vi "Begin.vi"() -> (0 "error out":errorcluster)   [LabVIEW 2013]
doc: "Called before other user functions, this VI is expected to open initial I/O refnums, load in file data, and do all program initialization. Notice that the <B>error out</B> terminal is simply used for data flow. Wiring it to other structures or subVIs ensures that this VI runs first."
uses:
  <vilib>/Rock Robotics/WPI/Joystick/WPI_JoystickDeviceEnum.ctl
  <vilib>/Rock Robotics/SystemInterfaces/Typedef/FPGA_TypedefDigitalModule.ctl
  <vilib>/Rock Robotics/SystemInterfaces/DIO/FPGA_DIOChannel.ctl
  <vilib>/Rock Robotics/SystemInterfaces/DIO/FPGA_DIORelayChannel.ctl
  <vilib>/Rock Robotics/SystemInterfaces/Typedef/FPGA_TypedefSolenoidModule.ctl
  <vilib>/Rock Robotics/WPI/Solenoid/WPI_SolenoidChannel.ctl
  <vilib>/Rock Robotics/WPI/Solenoid/WPI_SolenoidValue.ctl
  <vilib>/Rock Robotics/SystemInterfaces/DIO/FPGA_DIOPWMChannel.ctl
  <vilib>/Rock Robotics/WPI/Encoder/WPI_EncoderType.ctl
  <vilib>/Rock Robotics/WPI/Solenoid/WPI_SolenoidOpenDouble.vi
  <vilib>/Rock Robotics/WPI/Solenoid/WPI_SolenoidSetEnum.vi
  <vilib>/Rock Robotics/WPI/Counter/WPI_CounterDigitalInputToDigitalSource.vi
  <vilib>/Rock Robotics/WPI/RobotDrive/WPI_RobotDriveOpen2MotorWithVictor.vi
  <vilib>/Rock Robotics/WPI/MotorControl/WPI_MotorControlOpen Victor.vi
  <vilib>/Rock Robotics/WPI/Compressor/WPI_CompressorGetSetRefNum.vi
  <vilib>/Rock Robotics/WPI/Camera/WPI_CameraImageSize.ctl
  <vilib>/Rock Robotics/WPI/Camera/WPI_CameraWhite Balance Values.ctl
  <vilib>/Rock Robotics/WPI/Camera/WPI_CameraExposure Values.ctl
  <vilib>/Rock Robotics/WPI/Camera/WPI_CameraFrameRate.ctl
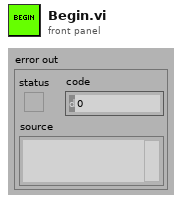
[diagram p1: front panel]
types:
  T1 = typedef "FPGA_DIOChannel.ctl" = enum8{"DIO 1", "DIO 2", "DIO 3", "DIO 4", "DIO 5", "DIO 6", "DIO 7", "DIO 8", "DIO 9", "DIO 10", "DIO 11", "DIO 12", "DIO 13", "DIO 14", "Invalid"}
  T2 = typedef "WPI_SolenoidChannel.ctl" = enum8{"Solenoid 1", "Solenoid 2", "Solenoid 3", "Solenoid 4", "Solenoid 5", "Solenoid 6", "Solenoid 7", "Solenoid 8", "Invalid"}
  T3 = typedef "FPGA_DIOPWMChannel.ctl" = enum8{"PWM 1", "PWM 2", "PWM 3", "PWM 4", "PWM 5", "PWM 6", "PWM 7", "PWM 8", "PWM 9", "PWM 10", "Invalid"}
  T4 = typedef "WPI_EncoderType.ctl" = enum16{"1x", "2x", "4x"}
  T5 = typedef "WPI_SolenoidValue.ctl" = enum16{"Off", "On", "Forward", "Reverse"}
  T6 = typedef "FPGA_TypedefSolenoidModule.ctl" = enum16{"Solenoid Module 1", "Solenoid Module 2"}
  T7 = typedef "FPGA_DIORelayChannel.ctl" = enum8{"Relay 1", "Relay 2", "Relay 3", "Relay 4", "Relay 5", "Relay 6", "Relay 7", "Relay 8", "Invalid"}
  T8 = typedef "WPI_JoystickDeviceEnum.ctl" = enum16{"USB 1", "USB 2", "USB 3", "USB 4", "Kinect 1", "Kinect 2"}
  T9 = typedef "FPGA_TypedefDigitalModule.ctl" = enum16{"Digital Module 1", "Digital Module 2"}
  T10 = typedef "WPI_CameraFrameRate.ctl" = u32
  T11 = typedef "WPI_CameraExposure Values.ctl" = enum16{"Auto", "Flicker-free 50 Hz", "Flicker-free 60 Hz", "Hold current"}
  T12 = typedef "WPI_CameraWhite Balance Values.ctl" = enum16{"Auto", "Fixed indoor", "Fixed outdoor 1", "Fixed outdoor 2", "Fixed fluorescent 1", "Fixed fluorescent 2", "Hold current"}
  T13 = typedef "WPI_CameraImageSize.ctl" = enum16{"640x480", "320x240", "160x120"}
  T14 = typedef "WPI_CameraDevRef.ctl" = cluster{"Camera Address":string, "CameraStatus":errorcluster, "Acquire Image Notifier":refnum<notifier>}
  T15 = typedef "WPI_DigitalInputDevRef.ctl" = cluster{"DevStatus":errorcluster, "DIO Channel":T1, "Digital Module":T9}
  T16 = typedef "WPI_MotorControlDeviceRef.ctl" = cluster{"DeviceStatus":errorcluster, "Type":enum16{"PWM", "CAN"}, "PWM":cluster{"Digital Module":T9, "PWM Channel":T3, "DeadBand":T17}, "CAN":cluster{"Device Number":u8, "Control Mode":T18, "Semaphore":T19, "Max Vout":dbl}, "Invert":bool, "TransformRef":T20, "InvTransformRef":T20}
  T17 = typedef "WPI_PWMDeadband.ctl" = cluster{"Name":string, "maxPositivePwm":i32, "minPositivePwm":i32, "centerPwm":i32, "maxNegativePwm":i32, "minNegativePwm":i32, "angularRange":u16}
  T18 = typedef "WPI_CANJaguar_ControlMode.ctl" = enum8{"Percent VBus", "Current", "Speed", "Position", "Voltage"}
  T19 = typedef "Semaphore RefNum" = refnum<k1>
  T20 = typedef "WPI_PWMTransform_ConPane.ctl" = refnum<vi>
  T21 = typedef "WPI_SolenoidDevRef.ctl" = cluster{"DevStatus":errorcluster, "Solenoid Module":T6, "Forward Solenoid Channel":T2, "Reverse Solenoid Channel":T2}
  T22 = typedef "FPGA_CounterEncoderSourceConvertionLVSourceType.ctl" = cluster{"DevStatus":errorcluster, "AnalogTriggerMode?":bool, "DigitalMode":cluster{"Digital Module":T9, "DIO Channel":T23}, "AnalogTriggerMode":cluster{"AnalogTriggerIndex":T24, "OutputType":T25}}
  T23 = typedef "FPGA_DIODigitalSourceChannel.ctl" = enum8{"DIO 1", "DIO 2", "DIO 3", "DIO 4", "DIO 5", "DIO 6", "DIO 7", "DIO 8", "DIO 9", "DIO 10", "DIO 11", "DIO 12", "DIO 13", "DIO 14", "Disabled"}
  T24 = typedef "FPGA_AnalogTriggerIndex.ctl" = enum8{"Trig 0", "Trig 1", "Trig 2", "Trig 3", "Trig 4", "Trig 5", "Trig 6", "Trig 7", "Invalid"}
  T25 = typedef "FPGA_AnalogTriggerOutType.ctl" = enum16{"InWindow", "TriggerState", "Rising", "Falling"}
  T26 = typedef "WPI_CompressorDevRef.ctl" = cluster{"DevStatus":errorcluster, "DigitalInputDevRef":T15, "RelayDevRef":T27}
  T27 = typedef "WPI_RelayDevRef.ctl" = cluster{"DevStatus":errorcluster, "Relay Channel":T7, "Digital Module":T9, "Relay Direction":T28}
  T28 = typedef "WPI_RelayDirection.ctl" = enum16{"Both directions", "Forward only", "Reverse only"}
  T29 = typedef "WPI_RobotDriveDevRef.ctl" = cluster{"DevStatus":errorcluster, "Motors[]":T16[], "Square Inputs":bool, "Max Output":dbl, "Isochronous":bool}
  T30 = typedef "WPI_EncoderDevRef.ctl" = cluster{"DevStatus":errorcluster, "EncoderIndex":T31, "CounterIndex":T32, "DistancePerCount":dbl, "Decoding Type":T4}
  T31 = typedef "FPGA_EncoderIdx.ctl" = enum8{"Enc 0", "Enc 1", "Enc 2", "Enc 3", "Invalid"}
  T32 = typedef "FPGA_CounterCtrSystemIndex.ctl" = enum8{"Ctr 0", "Ctr 1", "Ctr 2", "Ctr 3", "Ctr 4", "Ctr 5", "Ctr 6", "Ctr 7", "Invalid"}
  T33 = typedef "WPI_JoystickDevRef.ctl" = cluster{"Device":T8}
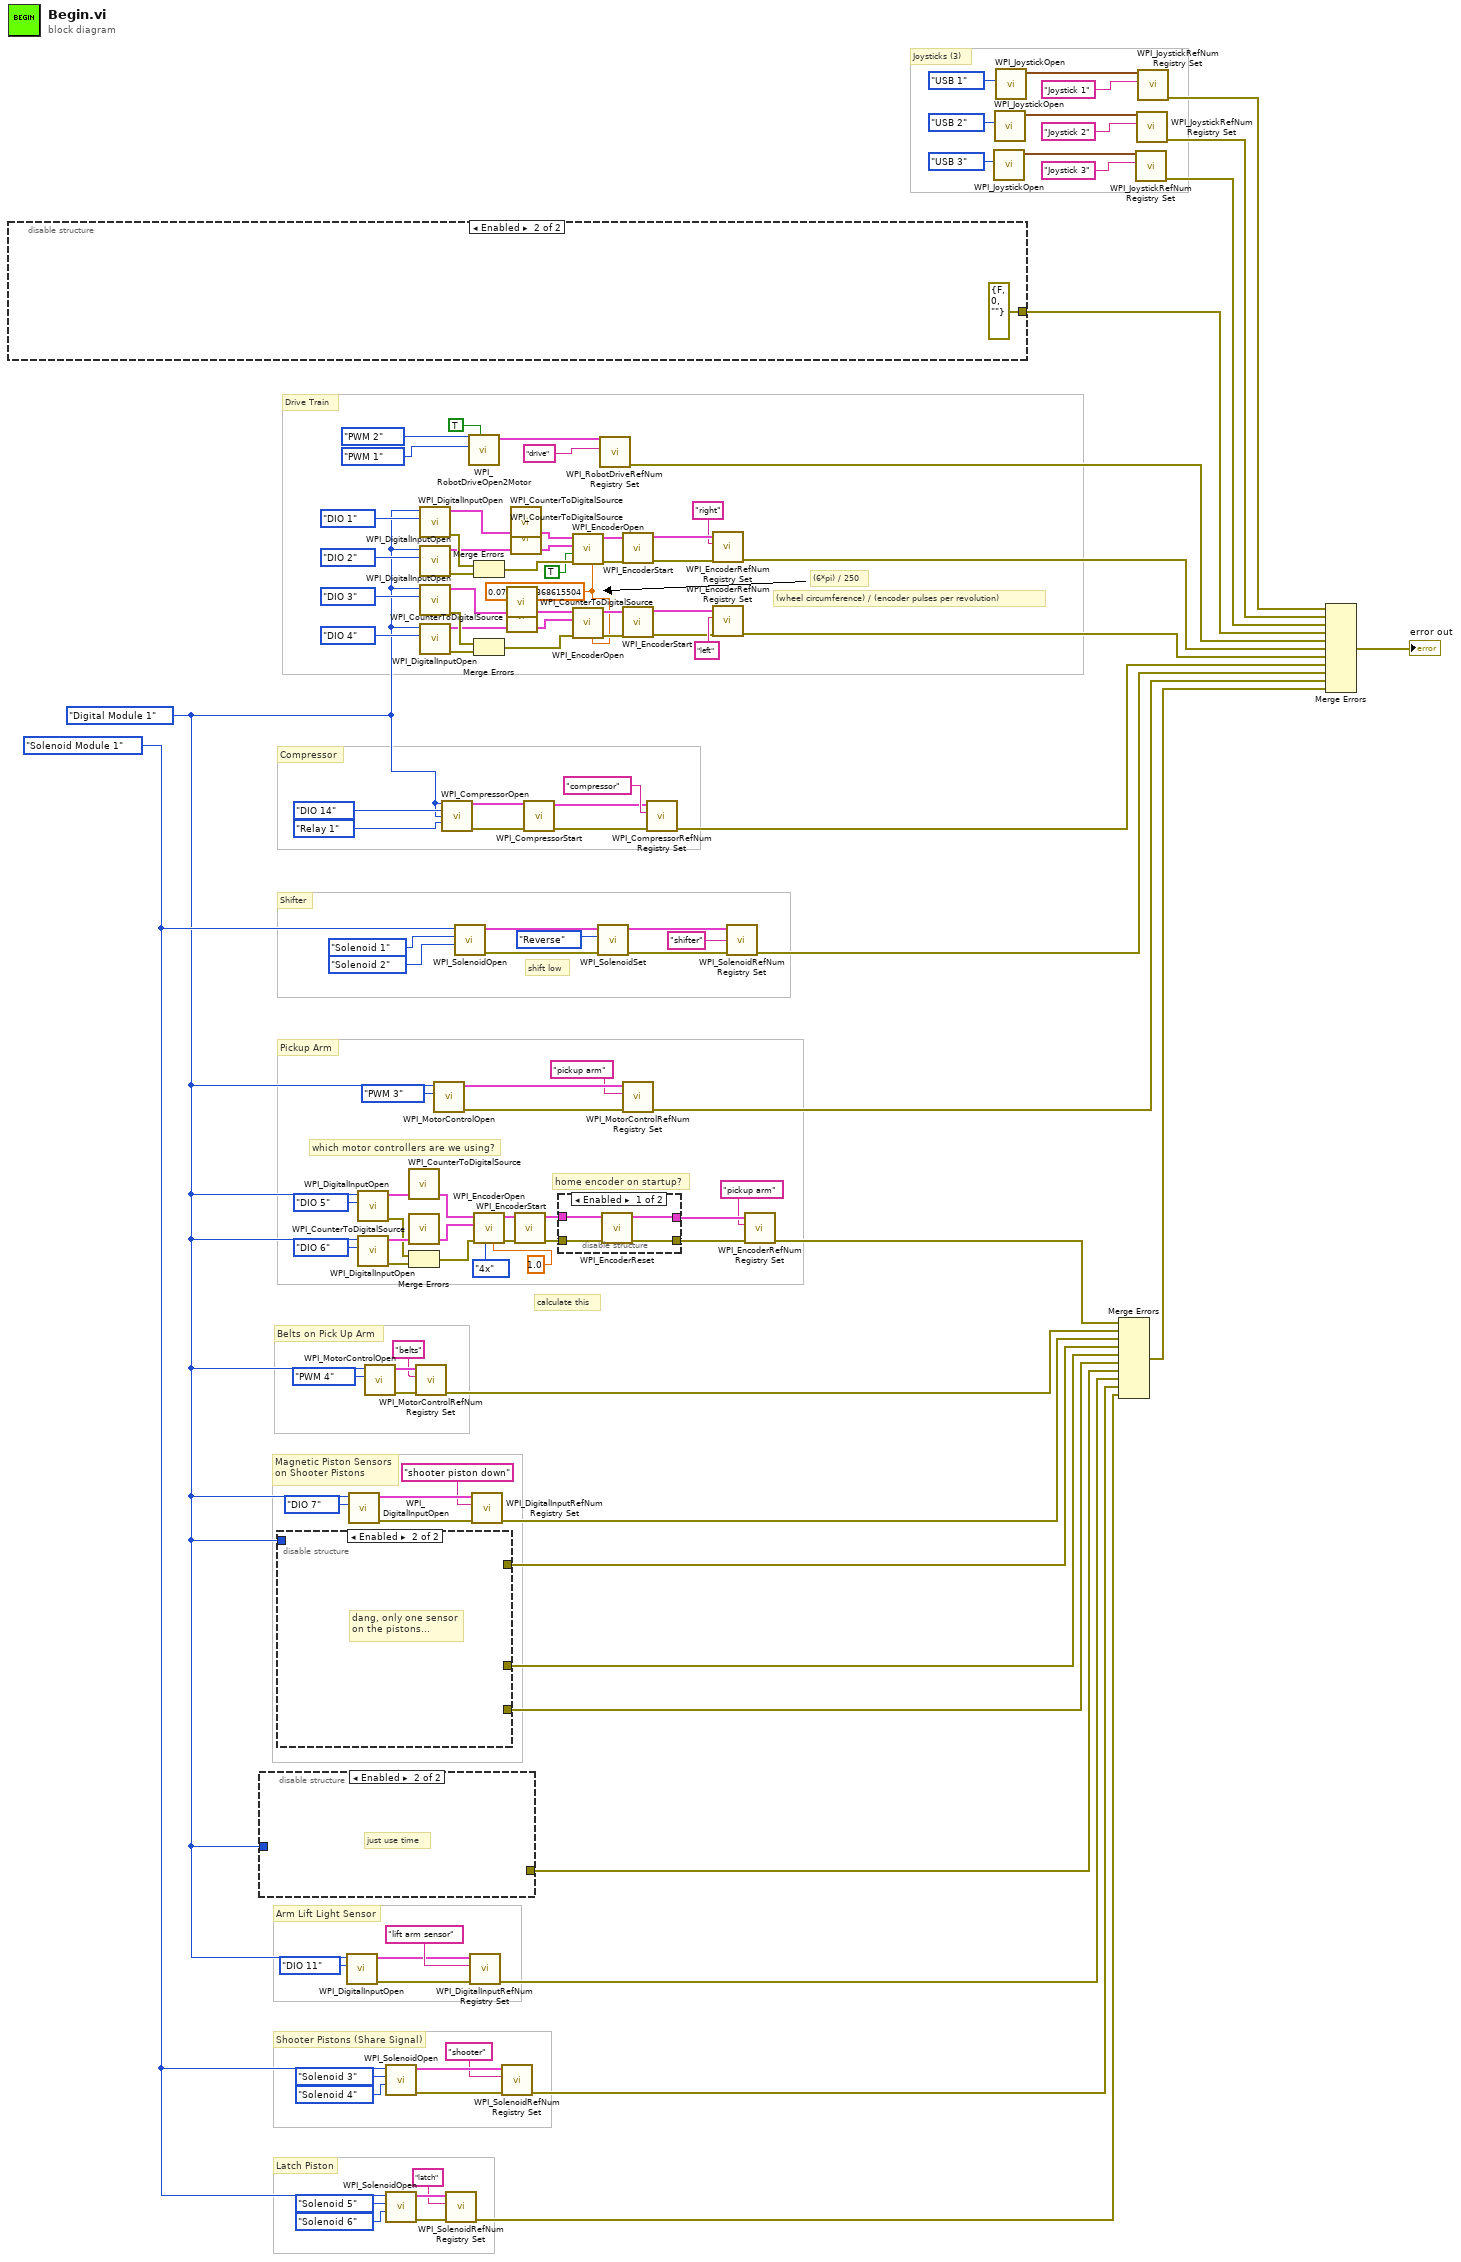
[diagram p0: block diagram]
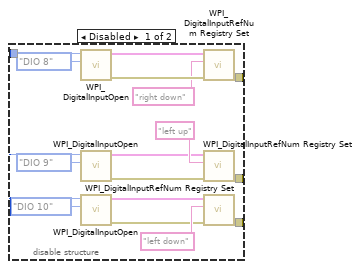
[diagram p2: hidden frame]
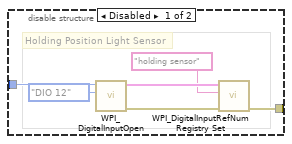
[diagram p3: hidden frame]
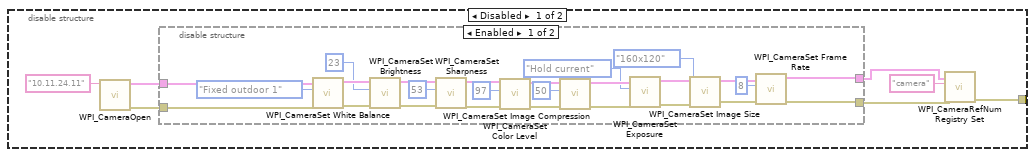
[diagram p5: hidden frame]
diagram:
  w71 = 0.07539822368615504 ("DistancePerCount")
  w12 = FPGA_TypedefSolenoidModule."Solenoid Module 1" ("Solenoid Module (Module 1)")
  w7 = FPGA_TypedefDigitalModule."Digital Module 1" ("Digital Module (Module 1)")
  # "Arm Lift Light Sensor"
  # "Joysticks (3)"
  # "Latch Piston"
  # "Shooter Pistons (Share Signal)"
  # "Magnetic Piston Sensors\non Shooter Pistons"
  # "Belts on Pick Up Arm"
  # "calculate this"
  # "Pickup Arm"
  # "home encoder on startup?"
  # "Shifter"
  # "Compressor"
  # "Drive Train"
  # "which motor controllers are we using?"
  # "shift low"
  # "(wheel circumference) / (encoder pulses per revolution)"
  # "(6*pi) / 250"
  n1 = disable-structure shown="Enabled" {
    disable-tunnel: [w128 errorcluster {"status"=FALSE, "code"=0, "source"=""} ("error out")] -> w115
    frame Disabled {
      n2 = call <vilib>:"WPI_CameraOpen.vi"("Camera Address"="10.11.24.11") -> ("error out"=w130:errorcluster, "CameraDevRef"=w132:T14)  [unwired: 9 in]
      n3 = disable-structure shown="Enabled" {
        disable-tunnel: w132 -> [w158 w162]
        disable-tunnel: [w136 w162] -> w131
        disable-tunnel: w130 -> [w145 w161]
        disable-tunnel: [w135 w161] -> w129
        frame Enabled {
          n4 = call <vilib>:"WPI_CameraSet White Balance.vi"("error in (no error)"=w145, "White Balance"=WPI_CameraWhite_Balance_Values."Fixed outdoor 1", "CameraDevRef"=w158) -> ("error out"=w146:errorcluster, "CameraDevRef Out"=w157:T14)  [unwired: 7 in]
          n5 = call <vilib>:"WPI_CameraSet Brightness.vi"("error in (no error)"=w146, "Brightness"=23, "CameraDevRef"=w157) -> ("error out"=w147:errorcluster, "CameraDevRef Out"=w156:T14)  [unwired: 7 in]
          n6 = call <vilib>:"WPI_CameraSet Sharpness.vi"("error in (no error)"=w147, "Sharpness"=53, "CameraDevRef"=w156) -> ("error out"=w148:errorcluster, "CameraDevRef Out"=w155:T14)  [unwired: 7 in]
          n7 = call <vilib>:"WPI_CameraSet Color Level.vi"("error in (no error)"=w148, "Color Level"=97, "CameraDevRef"=w155) -> ("error out"=w149:errorcluster, "CameraDevRef Out"=w154:T14)  [unwired: 7 in]
          n8 = call <vilib>:"WPI_CameraSet Image Compression.vi"("error in (no error)"=w149, "Compression"=50, "CameraDevRef"=w154) -> ("error out"=w160:errorcluster, "CameraDevRef Out"=w159:T14)  [unwired: 7 in]
          n9 = call <vilib>:"WPI_CameraSet Exposure.vi"("error in (no error)"=w160, "Exposure"=WPI_CameraExposure_Values."Hold current", "CameraDevRef"=w159) -> ("error out"=w150:errorcluster, "CameraDevRef Out"=w153:T14)  [unwired: 7 in]
          n10 = call <vilib>:"WPI_CameraSet Image Size.vi"("error in (no error)"=w150, "Image Size"=WPI_CameraImageSize."160x120", "CameraDevRef"=w153) -> ("error out"=w151:errorcluster, "CameraDevRef Out"=w152:T14)  [unwired: 7 in]
          n11 = call <vilib>:"WPI_CameraSet Frame Rate.vi"("error in (no error)"=w151, "Frame Rate (fps)"=T10 8, "CameraDevRef"=w152) -> ("error out"=w135:errorcluster, "CameraDevRef Out"=w136:T14)  [unwired: 7 in]
        }
        frame Disabled {
        }
      }
      n12 = call <vilib>:"WPI_CameraRefNum Registry Set.vi"("error in (no error)"=w129, "refnum name"="camera", "CameraDevRef"=w131) -> ("error out"=w128:errorcluster)  [unwired: 7 in, 1 out]
    }
    frame Enabled {
    }
  }
  n13 = disable-structure shown="Enabled" {
    disable-tunnel: w7 -> [w165 _]
    disable-tunnel: [w164 _] -> w3
    frame Disabled {
      # "Holding Position Light Sensor"
      n14 = call <vilib>:"WPI_DigitalInputOpen.vi"("DIO Channel"=FPGA_DIOChannel."DIO 12", "Digital Module (Module 1)"=w165) -> ("error out"=w168:errorcluster, "DigitalInputDevRef"=w167:T15)  [unwired: 8 in]
      n15 = call <vilib>:"WPI_DigitalInputRefNum Registry Set.vi"("error in (no error)"=w168, "refnum name"="holding sensor", "DigitalInputDevRef"=w167) -> ("error out"=w164:errorcluster)  [unwired: 7 in, 1 out]
    }
    frame Enabled {
      # "just use time"
    }
  }
  n16 = disable-structure shown="Enabled" {
    disable-tunnel: [w182 _] -> w23
    disable-tunnel: w7 -> [w172 _]
    disable-tunnel: [w171 _] -> w2
    disable-tunnel: [w170 _] -> w1
    frame Disabled {
      n17 = call <vilib>:"WPI_DigitalInputOpen.vi"("DIO Channel"=FPGA_DIOChannel."DIO 8", "Digital Module (Module 1)"=w172) -> ("error out"=w185:errorcluster, "DigitalInputDevRef"=w184:T15)  [unwired: 8 in]
      n18 = call <vilib>:"WPI_DigitalInputOpen.vi"("DIO Channel"=FPGA_DIOChannel."DIO 9", "Digital Module (Module 1)"=w172) -> ("error out"=w173:errorcluster, "DigitalInputDevRef"=w174:T15)  [unwired: 8 in]
      n19 = call <vilib>:"WPI_DigitalInputOpen.vi"("DIO Channel"=FPGA_DIOChannel."DIO 10", "Digital Module (Module 1)"=w172) -> ("error out"=w175:errorcluster, "DigitalInputDevRef"=w176:T15)  [unwired: 8 in]
      n20 = call <vilib>:"WPI_DigitalInputRefNum Registry Set.vi"("error in (no error)"=w185, "refnum name"="right down", "DigitalInputDevRef"=w184) -> ("error out"=w182:errorcluster)  [unwired: 7 in, 1 out]
      n21 = call <vilib>:"WPI_DigitalInputRefNum Registry Set.vi"("error in (no error)"=w173, "refnum name"="left up", "DigitalInputDevRef"=w174) -> ("error out"=w171:errorcluster)  [unwired: 7 in, 1 out]
      n22 = call <vilib>:"WPI_DigitalInputRefNum Registry Set.vi"("error in (no error)"=w175, "refnum name"="left down", "DigitalInputDevRef"=w176) -> ("error out"=w170:errorcluster)  [unwired: 7 in, 1 out]
    }
    frame Enabled {
      # "dang, only one sensor\non the pistons..."
    }
  }
  n23 = call <vilib>:"WPI_DigitalInputOpen.vi"("DIO Channel"=FPGA_DIOChannel."DIO 11", "Digital Module (Module 1)"=w7) -> ("error out"=w9:errorcluster, "DigitalInputDevRef"=w10:T15)  [unwired: 8 in]
  n24 = call <vilib>:"WPI_DigitalInputOpen.vi"("DIO Channel"=FPGA_DIOChannel."DIO 7", "Digital Module (Module 1)"=w7) -> ("error out"=w28:errorcluster, "DigitalInputDevRef"=w27:T15)  [unwired: 8 in]
  n25 = call <vilib>:"WPI_DigitalInputOpen.vi"("DIO Channel"=FPGA_DIOChannel."DIO 5", "Digital Module (Module 1)"=w7) -> ("error out"=w46:errorcluster, "DigitalInputDevRef"=w51:T15)  [unwired: 8 in]
  n26 = call <vilib>:"WPI_DigitalInputOpen.vi"("DIO Channel"=FPGA_DIOChannel."DIO 6", "Digital Module (Module 1)"=w7) -> ("error out"=w47:errorcluster, "DigitalInputDevRef"=w50:T15)  [unwired: 8 in]
  n27 = call-poly <vilib>:"WPI_MotorControlOpen.vi"("PWM Channel"=FPGA_DIOPWMChannel."PWM 4", "Digital Module (Module 1)"=w7) -> ("error out"=w34:errorcluster, "MotorControlDeviceRef"=w33:T16)  [unwired: 8 in]
  n28 = call-poly <vilib>:"WPI_SolenoidOpen.vi"("Reverse Solenoid Channel"=WPI_SolenoidChannel."Solenoid 4", "Forward Solenoid Channel"=WPI_SolenoidChannel."Solenoid 3", "Solenoid Module (Module 1)"=w12) -> ("error out"=w18:errorcluster, "SolenoidDevRef"=w17:T21)  [unwired: 7 in]
  n29 = call-poly <vilib>:"WPI_SolenoidOpen.vi"("Reverse Solenoid Channel"=WPI_SolenoidChannel."Solenoid 6", "Forward Solenoid Channel"=WPI_SolenoidChannel."Solenoid 5", "Solenoid Module (Module 1)"=w12) -> ("error out"=w16:errorcluster, "SolenoidDevRef"=w15:T21)  [unwired: 7 in]
  n30 = call-poly <vilib>:"WPI_CounterToDigitalSource.vi"("DigitalInputDevRef"=w51) -> ("Digital Source"=w49:T22)  [unwired: 6 in]
  n31 = call-poly <vilib>:"WPI_CounterToDigitalSource.vi"("DigitalInputDevRef"=w50) -> ("Digital Source"=w48:T22)  [unwired: 6 in]
  n32 = Merge Errors(w46, w47) -> (w45:errorcluster)
  n33 = call <vilib>:"WPI_MotorControlRefNum Registry Set.vi"("error in (no error)"=w34, "refnum name"="belts", "MotorControlDevRef"=w33) -> ("error out"=w31:errorcluster)  [unwired: 7 in, 1 out]
  n34 = call <vilib>:"WPI_DigitalInputOpen.vi"("DIO Channel"=FPGA_DIOChannel."DIO 1", "Digital Module (Module 1)"=w7) -> ("error out"=w65:errorcluster, "DigitalInputDevRef"=w79:T15)  [unwired: 8 in]
  n35 = call <vilib>:"WPI_DigitalInputOpen.vi"("DIO Channel"=FPGA_DIOChannel."DIO 2", "Digital Module (Module 1)"=w7) -> ("error out"=w67:errorcluster, "DigitalInputDevRef"=w64:T15)  [unwired: 8 in]
  n36 = call <vilib>:"WPI_DigitalInputOpen.vi"("DIO Channel"=FPGA_DIOChannel."DIO 3", "Digital Module (Module 1)"=w7) -> ("error out"=w68:errorcluster, "DigitalInputDevRef"=w93:T15)  [unwired: 8 in]
  n37 = call <vilib>:"WPI_DigitalInputOpen.vi"("DIO Channel"=FPGA_DIOChannel."DIO 4", "Digital Module (Module 1)"=w7) -> ("error out"=w70:errorcluster, "DigitalInputDevRef"=w63:T15)  [unwired: 8 in]
  n38 = call-poly <vilib>:"WPI_MotorControlOpen.vi"("PWM Channel"=FPGA_DIOPWMChannel."PWM 3", "Digital Module (Module 1)"=w7) -> ("error out"=w58:errorcluster, "MotorControlDeviceRef"=w57:T16)  [unwired: 8 in]
  n39 = call <vilib>:"WPI_CompressorOpen.vi"("Pressure Switch Digital Module (Module 1)"=w7, "Pressure Switch DIO Channel"=FPGA_DIOChannel."DIO 14", "Relay Digital Module (Module 1)"=w7, "Relay Channel"=FPGA_DIORelayChannel."Relay 1") -> ("CompressorDevRef"=w107:T26, "error out"=w106:errorcluster)  [unwired: 10 in]
  n40 = call <vilib>:"WPI_SolenoidRefNum Registry Set.vi"("error in (no error)"=w16, "refnum name"="latch", "SolenoidDevRef"=w15) -> ("error out"=w6:errorcluster)  [unwired: 7 in, 1 out]
  n41 = call-poly <vilib>:"WPI_SolenoidOpen.vi"("Reverse Solenoid Channel"=WPI_SolenoidChannel."Solenoid 2", "Forward Solenoid Channel"=WPI_SolenoidChannel."Solenoid 1", "Solenoid Module (Module 1)"=w12) -> ("error out"=w98:errorcluster, "SolenoidDevRef"=w99:T21)  [unwired: 7 in]
  n42 = call-poly <vilib>:"WPI_RobotDriveOpen2Motor.vi"("Left Motor Inverted"=TRUE, "Right Motor"=FPGA_DIOPWMChannel."PWM 1", "Left Motor"=FPGA_DIOPWMChannel."PWM 2") -> ("RobotDriveDevRef"=w95:T29)  [unwired: 7 in, 1 out]
  n43 = call <vilib>:"WPI_DigitalInputRefNum Registry Set.vi"("error in (no error)"=w9, "refnum name"="lift arm sensor", "DigitalInputDevRef"=w10) -> ("error out"=w4:errorcluster)  [unwired: 7 in, 1 out]
  n44 = call <vilib>:"WPI_DigitalInputRefNum Registry Set.vi"("error in (no error)"=w28, "refnum name"="shooter piston down", "DigitalInputDevRef"=w27) -> ("error out"=w24:errorcluster)  [unwired: 7 in, 1 out]
  n45 = Merge Errors(w65, w67) -> (w66:errorcluster)
  n46 = Merge Errors(w68, w70) -> (w69:errorcluster)
  n47 = call <vilib>:"WPI_EncoderOpen.vi"("DistancePerCount"=1.0, "Decoding Type"=WPI_EncoderType."4x", "error in (no error)"=w45, "BSource"=w48, "ASource"=w49) -> ("error out"=w44:errorcluster, "EncoderDevRef"=w43:T30)  [unwired: 5 in]
  n48 = call <vilib>:"WPI_SolenoidRefNum Registry Set.vi"("error in (no error)"=w18, "refnum name"="shooter", "SolenoidDevRef"=w17) -> ("error out"=w5:errorcluster)  [unwired: 7 in, 1 out]
  n49 = call-poly <vilib>:"WPI_CounterToDigitalSource.vi"("DigitalInputDevRef"=w93) -> ("Digital Source"=w86:T22)  [unwired: 6 in]
  n50 = call-poly <vilib>:"WPI_CounterToDigitalSource.vi"("DigitalInputDevRef"=w63) -> ("Digital Source"=w87:T22)  [unwired: 6 in]
  n51 = call-poly <vilib>:"WPI_CounterToDigitalSource.vi"("DigitalInputDevRef"=w79) -> ("Digital Source"=w85:T22)  [unwired: 6 in]
  n52 = call-poly <vilib>:"WPI_CounterToDigitalSource.vi"("DigitalInputDevRef"=w64) -> ("Digital Source"=w84:T22)  [unwired: 6 in]
  n53 = call <vilib>:"WPI_EncoderStart.vi"("error in (no error)"=w44, "EncoderDevRef"=w43) -> ("error out"=w42:errorcluster, "EncoderDevRef"=w41:T30)  [unwired: 8 in]
  n54 = call <vilib>:"WPI_CompressorStart.vi"("error in (no error)"=w106, "CompressorDevRef"=w107) -> ("error out"=w105:errorcluster, "CompressorDevRef"=w104:T26)  [unwired: 8 in]
  n55 = disable-structure shown="Enabled" {
    disable-tunnel: w42 -> [w189 w190]
    disable-tunnel: w41 -> [w188 w191]
    disable-tunnel: [w187 w191] -> w39
    disable-tunnel: [w186 w190] -> w40
    frame Enabled {
      n56 = call <vilib>:"WPI_EncoderReset.vi"("error in (no error)"=w189, "EncoderDevRef"=w188) -> ("error out"=w186:errorcluster, "EncoderDevRef"=w187:T30)  [unwired: 8 in]
    }
    frame Disabled {
    }
  }
  n57 = call <vilib>:"WPI_EncoderOpen.vi"("DistancePerCount"=w71, "error in (no error)"=w66, "Invert Direction (False)"=TRUE, "BSource"=w84, "ASource"=w85) -> ("error out"=w83:errorcluster, "EncoderDevRef"=w82:T30)  [unwired: 5 in]
  n58 = call <vilib>:"WPI_EncoderOpen.vi"("DistancePerCount"=w71, "error in (no error)"=w69, "BSource"=w87, "ASource"=w86) -> ("error out"=w88:errorcluster, "EncoderDevRef"=w89:T30)  [unwired: 6 in]
  n59 = call-poly <vilib>:"WPI_SolenoidSet.vi"("error in (no error)"=w98, "Value"=WPI_SolenoidValue."Reverse", "SolenoidDevRef"=w99) -> ("error out"=w97:errorcluster, "SolenoidDevRef"=w96:T21)  [unwired: 7 in]
  n60 = call <vilib>:"WPI_RobotDriveRefNum Registry Set.vi"("refnum name"="drive", "RobotDriveDevRef"=w95) -> ("error out"=w114:errorcluster)  [unwired: 8 in, 1 out]
  n61 = call <vilib>:"WPI_EncoderStart.vi"("error in (no error)"=w83, "EncoderDevRef"=w82) -> ("error out"=w81:errorcluster, "EncoderDevRef"=w80:T30)  [unwired: 8 in]
  n62 = call <vilib>:"WPI_EncoderStart.vi"("error in (no error)"=w88, "EncoderDevRef"=w89) -> ("error out"=w90:errorcluster, "EncoderDevRef"=w91:T30)  [unwired: 8 in]
  n63 = call <vilib>:"WPI_MotorControlRefNum Registry Set.vi"("error in (no error)"=w58, "refnum name"="pickup arm", "MotorControlDevRef"=w57) -> ("error out"=w54:errorcluster)  [unwired: 7 in, 1 out]
  n64 = call <vilib>:"WPI_CompressorRefNum Registry Set.vi"("error in (no error)"=w105, "refnum name"="compressor", "CompressorDevRef"=w104) -> ("error out"=w59:errorcluster)  [unwired: 7 in, 1 out]
  n65 = call <vilib>:"WPI_EncoderRefNum Registry Set.vi"("error in (no error)"=w81, "refnum name"="right", "EncoderDevRef"=w80) -> ("error out"=w113:errorcluster)  [unwired: 7 in, 1 out]
  n66 = call <vilib>:"WPI_EncoderRefNum Registry Set.vi"("error in (no error)"=w90, "refnum name"="left", "EncoderDevRef"=w91) -> ("error out"=w112:errorcluster)  [unwired: 7 in, 1 out]
  n67 = call <vilib>:"WPI_SolenoidRefNum Registry Set.vi"("error in (no error)"=w97, "refnum name"="shifter", "SolenoidDevRef"=w96) -> ("error out"=w60:errorcluster)  [unwired: 7 in, 1 out]
  n68 = call <vilib>:"WPI_EncoderRefNum Registry Set.vi"("error in (no error)"=w40, "refnum name"="pickup arm", "EncoderDevRef"=w39) -> ("error out"=w30:errorcluster)  [unwired: 7 in, 1 out]
  n69 = call <vilib>:"WPI_JoystickOpen.vi"("JoystickDevice"=WPI_JoystickDeviceEnum."USB 3") -> ("JoystickDevRef"=w126:T33)  [unwired: 10 in]
  n70 = call <vilib>:"WPI_JoystickOpen.vi"("JoystickDevice"=WPI_JoystickDeviceEnum."USB 2") -> ("JoystickDevRef"=w123:T33)  [unwired: 10 in]
  n71 = call <vilib>:"WPI_JoystickOpen.vi"("JoystickDevice"=WPI_JoystickDeviceEnum."USB 1") -> ("JoystickDevRef"=w120:T33)  [unwired: 10 in]
  n72 = Merge Errors(w30, w31, w24, w23, w2, w1, w3, w4, w5, w6) -> (w29:errorcluster)
  n73 = call <vilib>:"WPI_JoystickRefNum Registry Set.vi"("refnum name"="Joystick 3", "JoystickDevRef"=w126) -> ("error out"=w116:errorcluster)  [unwired: 8 in, 1 out]
  n74 = call <vilib>:"WPI_JoystickRefNum Registry Set.vi"("refnum name"="Joystick 2", "JoystickDevRef"=w123) -> ("error out"=w117:errorcluster)  [unwired: 8 in, 1 out]
  n75 = call <vilib>:"WPI_JoystickRefNum Registry Set.vi"("refnum name"="Joystick 1", "JoystickDevRef"=w120) -> ("error out"=w118:errorcluster)  [unwired: 8 in, 1 out]
  n76 = Merge Errors(w118, w117, w116, w115, w114, w113, w112, w59, w60, w54, w29) -> (→"error out":errorcluster)
